vi "FT-IR Parameter Laden-Speichern.vi"(0 "NoOfGases In":u32, 1 "CurrentRecipe In":string, 2 "labEnabled In":bool, 3 "labPath In":path, 4 "labBaseName In":string, 5 "NoOfScan In":u32, 8 "Aktion":T1) -> (12 "NoOfGases":u32, 14 "CurrentRecipe":string, 15 "labEnabled":bool, 16 "labPath":path, 17 "labBaseName":string, 18 "NoOfScan":u32)   [LabVIEW 2020, in "FT-IR.lvlib"]
uses:
  FT-IR.lvlib
  Aktionen Parameter Laden-Speichern.ctl
  FGV FT-IR Diagnose Aktionen.ctl
  <vilib>/Utility/config.llb/Read Key (U32).vi
  <vilib>/Utility/config.llb/Read Key (String).vi
  <vilib>/Utility/config.llb/Read Key (Boolean).vi
  <vilib>/Utility/config.llb/Read Key (Path).vi
  <vilib>/Utility/config.llb/Read Key (Double).vi
  <vilib>/Utility/config.llb/Write Key (U32).vi
  <vilib>/Utility/config.llb/Write Key (String).vi
  <vilib>/Utility/config.llb/Write Key (Boolean).vi
  <vilib>/Utility/config.llb/Write Key (Path).vi
  <vilib>/Utility/config.llb/Write Key (Double).vi
  <vilib>/Utility/config.llb/NI_LVConfig.lvlib
  Allgemein/allgemeine Sub-VIs.lvlib
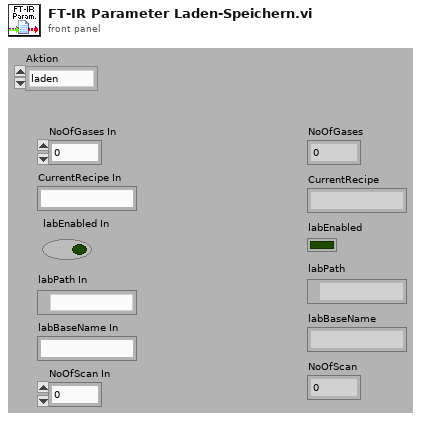
[diagram p1: front panel]
types:
  T1 = typedef "FT-IR.lvlib/Aktionen Parameter Laden-Speichern.ctl" = enum16{"laden", "speichern"}
  T2 = typedef "NI_LVConfig.lvlib/Config Data RefNum.ctl" = refnum<k1>
  T3 = typedef "FT-IR.lvlib/FGV FT-IR Diagnose Aktionen.ctl" = enum16{"Lesen", "Diagnose Schreiben", "Min Schreiben", "Max Schreiben"}
  T4 = cluster{"LaserPP Max":dbl, "LinCheck Max":dbl, "sBeam Max":dbl}
  T5 = cluster{"LaserPP Min":dbl, "LinCheck Min":dbl, "sBeam Min":dbl}
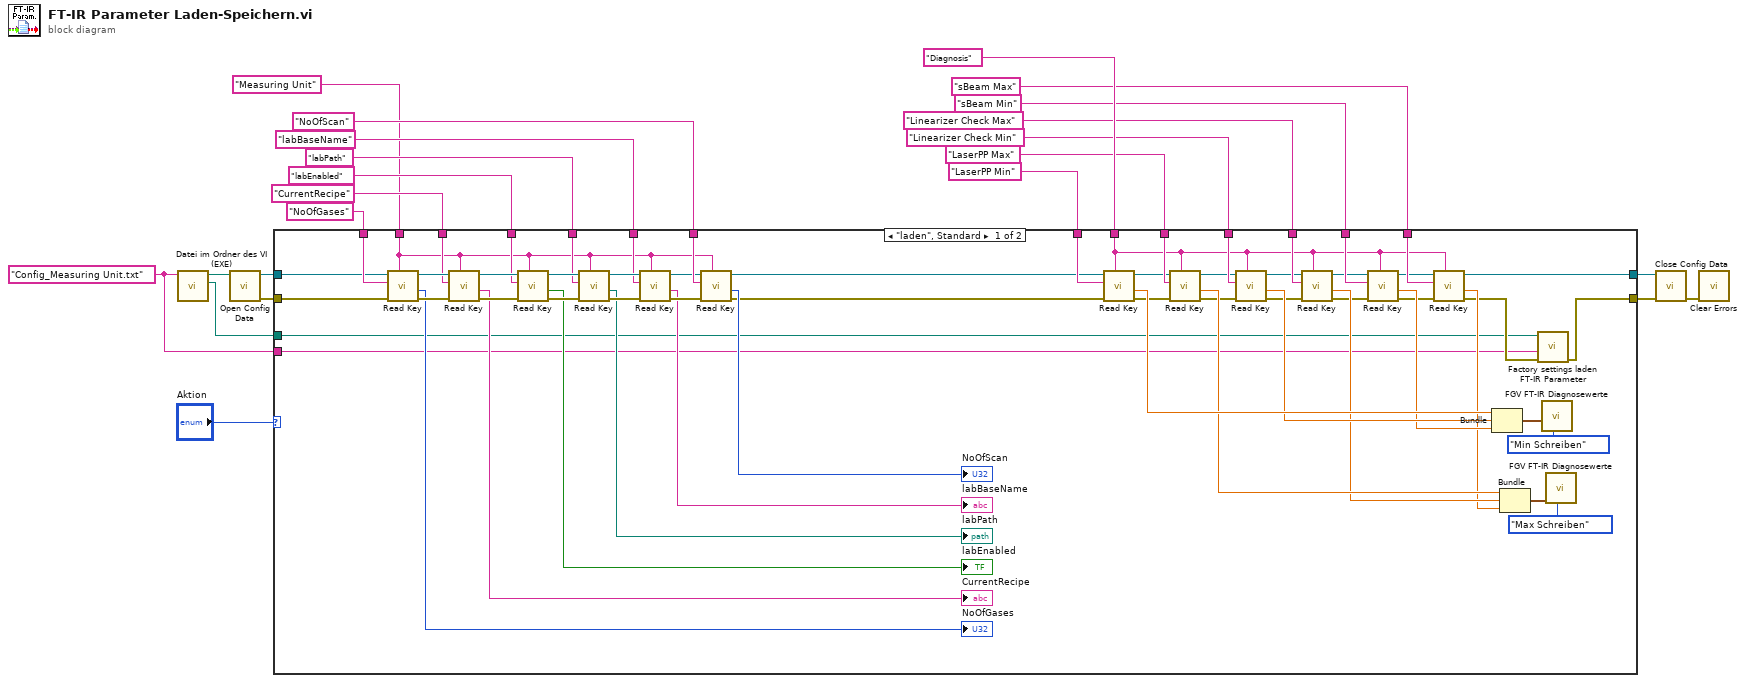
[diagram p0: block diagram]
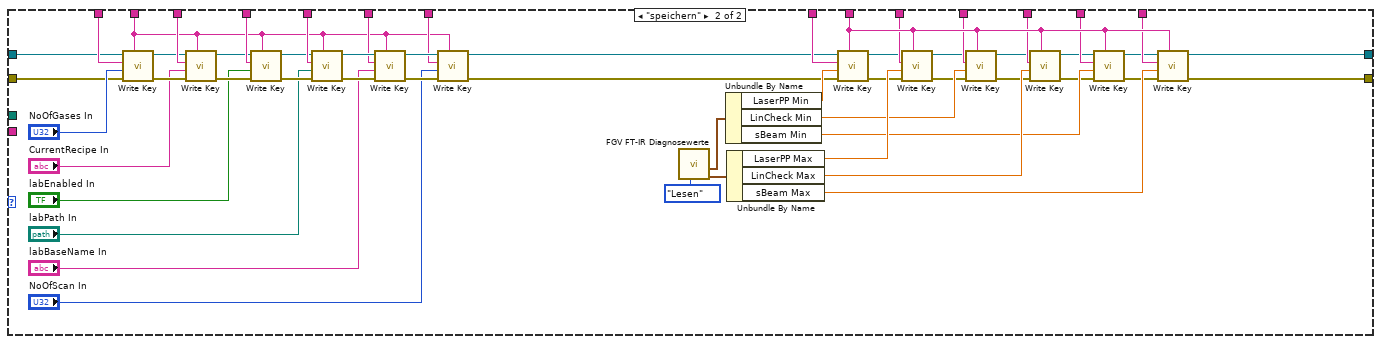
[diagram p2: hidden frame]
diagram:
  w1 = "Config_Measuring Unit.txt" ("Dateiname")
  n1 = call "Datei im Ordner des VI (EXE).vi"("Dateiname"=w1) -> ("Ordner des Haupt-VIs"=w2:path, "Dateipfad im Ordner des Haupt-VIs"=w23:path)  [unwired: 8 in, 1 out]
  n2 = call <vilib>:"Open Config Data.vi"("configuration file path"=w23) -> ("error out"=w17:errorcluster, "refnum"=w18:T2)  [unwired: 8 in, 1 out]
  n3 = case shown="\"laden\", Standard" "Aktion" {
    tunnel: [w24 w86] -> w22
    tunnel: [w36 w87] -> w21
    tunnel: "NoOfScan" ("key") -> [w82 w119]
    tunnel: "NoOfGases" ("key") -> [w81 w137]
    tunnel: w18 -> [w72 w125]
    tunnel: w17 -> [w71 w124]
    tunnel: "CurrentRecipe" ("key") -> [w70 w135]
    tunnel: "labEnabled" ("key") -> [w69 w134]
    tunnel: "labPath" ("key") -> [w68 w133]
    tunnel: "labBaseName" ("key") -> [w67 w120]
    tunnel: "Measuring Unit" ("section") -> [w30 w85]
    tunnel: "Diagnosis" ("section") -> [w49 w113]
    tunnel: "sBeam Max" ("key") -> [w54 w112]
    tunnel: "sBeam Min" ("key") -> [w53 w111]
    tunnel: "Linearizer Check Max" ("key") -> [w52 w110]
    tunnel: "Linearizer Check Min" ("key") -> [w51 w109]
    tunnel: "LaserPP Max" ("key") -> [w50 w108]
    tunnel: "LaserPP Min" ("key") -> [w56 w107]
    tunnel: w2 -> [w26 _]
    tunnel: w1 -> [w25 _]
    frame "laden", Default {
      n4 = call-poly <vilib>:"Read Key.vi"("section"=w30, "error in (no error)"=w71, "key"=w81, "refnum"=w72) -> ("error out"=w80:errorcluster, "value"=→"NoOfGases":u32, "refnum out"=w79:T2)  [unwired: 4 in, 1 out]
      n5 = call-poly <vilib>:"Read Key.vi"("section"=w30, "error in (no error)"=w80, "key"=w70, "refnum"=w79) -> ("error out"=w78:errorcluster, "value"=→"CurrentRecipe":string, "refnum out"=w77:T2)  [unwired: 4 in, 1 out]
      n6 = call-poly <vilib>:"Read Key.vi"("section"=w30, "error in (no error)"=w78, "key"=w69, "refnum"=w77) -> ("error out"=w76:errorcluster, "value"=→"labEnabled":bool, "refnum out"=w75:T2)  [unwired: 4 in, 1 out]
      n7 = call-poly <vilib>:"Read Key.vi"("section"=w30, "error in (no error)"=w76, "key"=w68, "refnum"=w75) -> ("error out"=w74:errorcluster, "value"=→"labPath":path, "refnum out"=w73:T2)  [unwired: 4 in, 1 out]
      n8 = call-poly <vilib>:"Read Key.vi"("section"=w30, "error in (no error)"=w74, "key"=w67, "refnum"=w73) -> ("error out"=w65:errorcluster, "value"=→"labBaseName":string, "refnum out"=w66:T2)  [unwired: 4 in, 1 out]
      n9 = call-poly <vilib>:"Read Key.vi"("section"=w30, "error in (no error)"=w65, "key"=w82, "refnum"=w66) -> ("error out"=w28:errorcluster, "value"=→"NoOfScan":u32, "refnum out"=w29:T2)  [unwired: 4 in, 1 out]
      n10 = call-poly <vilib>:"Read Key.vi"("section"=w49, "error in (no error)"=w28, "key"=w56, "refnum"=w29) -> ("error out"=w35:errorcluster, "value"=w55:dbl, "refnum out"=w41:T2)  [unwired: 4 in, 1 out]
      n11 = call-poly <vilib>:"Read Key.vi"("section"=w49, "error in (no error)"=w35, "key"=w50, "refnum"=w41) -> ("error out"=w34:errorcluster, "value"=w45:dbl, "refnum out"=w40:T2)  [unwired: 4 in, 1 out]
      n12 = call-poly <vilib>:"Read Key.vi"("section"=w49, "error in (no error)"=w34, "key"=w51, "refnum"=w40) -> ("error out"=w33:errorcluster, "value"=w47:dbl, "refnum out"=w39:T2)  [unwired: 4 in, 1 out]
      n13 = call-poly <vilib>:"Read Key.vi"("section"=w49, "error in (no error)"=w33, "key"=w52, "refnum"=w39) -> ("error out"=w32:errorcluster, "value"=w44:dbl, "refnum out"=w38:T2)  [unwired: 4 in, 1 out]
      n14 = call-poly <vilib>:"Read Key.vi"("section"=w49, "error in (no error)"=w32, "key"=w53, "refnum"=w38) -> ("error out"=w31:errorcluster, "value"=w46:dbl, "refnum out"=w37:T2)  [unwired: 4 in, 1 out]
      n15 = call-poly <vilib>:"Read Key.vi"("section"=w49, "error in (no error)"=w31, "key"=w54, "refnum"=w37) -> ("error out"=w27:errorcluster, "value"=w43:dbl, "refnum out"=w36:T2)  [unwired: 4 in, 1 out]
      n16 = Bundle("value"=w55, "value"=w47, "value"=w46) -> (w48:cluster{"value":dbl, "value":dbl, "value":dbl})  [unwired: 1 in]
      n17 = Bundle("value"=w45, "value"=w44, "value"=w43) -> (w42:cluster{"value":dbl, "value":dbl, "value":dbl})  [unwired: 1 in]
      n18 = call "Factory settings laden FT-IR Parameter.vi"("error in (no error)"=w27, "Dateiname"=w25, "Ordner des Haupt-VIs"=w26) -> ("error out"=w24:errorcluster)  [unwired: 8 in]
      n19 = call "FGV FT-IR Diagnosewerte.vi"("Aktionen"=FGV_FT-IR_Diagnose_Aktionen."Min Schreiben", "FT-IR MIN"=w48) -> ()  [unwired: 4 in, 6 out]
      n20 = call "FGV FT-IR Diagnosewerte.vi"("Aktionen"=FGV_FT-IR_Diagnose_Aktionen."Max Schreiben", "FT-IR MAX"=w42) -> ()  [unwired: 4 in, 6 out]
    }
    frame "speichern" {
      n21 = call-poly <vilib>:"Write Key.vi"("section"=w85, "error in (no error)"=w124, "value"="NoOfGases In", "key"=w137, "refnum"=w125) -> ("error out"=w123:errorcluster, "refnum out"=w128:T2)  [unwired: 4 in, 1 out]
      n22 = call-poly <vilib>:"Write Key.vi"("section"=w85, "error in (no error)"=w123, "value"="CurrentRecipe In", "key"=w135, "refnum"=w128) -> ("error out"=w122:errorcluster, "refnum out"=w127:T2)  [unwired: 4 in, 1 out]
      n23 = call-poly <vilib>:"Write Key.vi"("section"=w85, "error in (no error)"=w122, "value"="labEnabled In", "key"=w134, "refnum"=w127) -> ("error out"=w121:errorcluster, "refnum out"=w126:T2)  [unwired: 4 in, 1 out]
      n24 = call-poly <vilib>:"Write Key.vi"("section"=w85, "error in (no error)"=w121, "value"="labPath In", "key"=w133, "refnum"=w126) -> ("error out"=w132:errorcluster, "refnum out"=w131:T2)  [unwired: 4 in, 1 out]
      n25 = call-poly <vilib>:"Write Key.vi"("section"=w85, "error in (no error)"=w132, "value"="labBaseName In", "key"=w120, "refnum"=w131) -> ("error out"=w130:errorcluster, "refnum out"=w129:T2)  [unwired: 4 in, 1 out]
      n26 = call-poly <vilib>:"Write Key.vi"("section"=w85, "error in (no error)"=w130, "value"="NoOfScan In", "key"=w119, "refnum"=w129) -> ("error out"=w83:errorcluster, "refnum out"=w84:T2)  [unwired: 4 in, 1 out]
      n27 = call "FGV FT-IR Diagnosewerte.vi"("Aktionen"=FGV_FT-IR_Diagnose_Aktionen."Lesen") -> ("FT-IR MAX"=w104:T4, "FT-IR MIN"=w105:T5)  [unwired: 5 in, 4 out]
      n28 = Unbundle By Name(w105) -> ("LaserPP Min"=w103:dbl, "LinCheck Min"=w101:dbl, "sBeam Min"=w99:dbl)
      n29 = Unbundle By Name(w104) -> ("LaserPP Max"=w102:dbl, "LinCheck Max"=w100:dbl, "sBeam Max"=w98:dbl)
      n30 = call-poly <vilib>:"Write Key.vi"("section"=w113, "error in (no error)"=w83, "value"=w103, "key"=w107, "refnum"=w84) -> ("error out"=w96:errorcluster, "refnum out"=w97:T2)  [unwired: 4 in, 1 out]
      n31 = call-poly <vilib>:"Write Key.vi"("section"=w113, "error in (no error)"=w96, "value"=w102, "key"=w108, "refnum"=w97) -> ("error out"=w94:errorcluster, "refnum out"=w95:T2)  [unwired: 4 in, 1 out]
      n32 = call-poly <vilib>:"Write Key.vi"("section"=w113, "error in (no error)"=w94, "value"=w101, "key"=w109, "refnum"=w95) -> ("error out"=w92:errorcluster, "refnum out"=w93:T2)  [unwired: 4 in, 1 out]
      n33 = call-poly <vilib>:"Write Key.vi"("section"=w113, "error in (no error)"=w92, "value"=w100, "key"=w110, "refnum"=w93) -> ("error out"=w90:errorcluster, "refnum out"=w91:T2)  [unwired: 4 in, 1 out]
      n34 = call-poly <vilib>:"Write Key.vi"("section"=w113, "error in (no error)"=w90, "value"=w99, "key"=w111, "refnum"=w91) -> ("error out"=w88:errorcluster, "refnum out"=w89:T2)  [unwired: 4 in, 1 out]
      n35 = call-poly <vilib>:"Write Key.vi"("section"=w113, "error in (no error)"=w88, "value"=w98, "key"=w112, "refnum"=w89) -> ("error out"=w86:errorcluster, "refnum out"=w87:T2)  [unwired: 4 in, 1 out]
    }
  }
  n36 = call <vilib>:"Close Config Data.vi"("error in (no error)"=w22, "refnum"=w21) -> ("error out"=w3:errorcluster)  [unwired: 8 in, 1 out]
  n37 = call <vilib>:"Clear Errors.vi"("error in (no error)"=w3) -> ()  [unwired: 5 in, 2 out]
